vi "Command_Goto.vi"(2 "node":string, 3 "Side":T1, 4 "Desired Position":sgl=100.0 min=0 max=100, 6 "error in":errorcluster) -> (5 "error out":errorcluster)   [LabVIEW 2012]
doc: "This will open or close the gripper to a specific position"
uses:
  <userlib>/ROSforLV/ROS/Code/SubVIs/BaxterSide.ctl
  <userlib>/ROSforLV/ROS/Code/Console/Servers/ServerSubs/TopicDef.ctl
  <userlib>/ROSforLV/ROS/Code/SubVIs/_ROSDirection.ctl
panel:
  # "Gripper position is from [0.0-100.0] [close-open]"
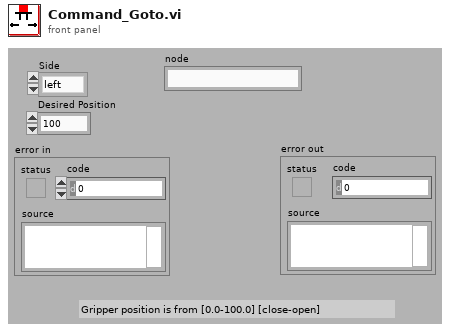
[diagram p1: front panel]
types:
  T1 = typedef "BaxterSide.ctl" = enum16{"left", "right"}
  T2 = typedef "TopicDef.ctl" = cluster{"Topic":string, "Type":string, "Action":T3, "Update (ms)":u16, "write queue":u16}
  T3 = typedef "_ROSDirection.ctl" = enum16{"Node", "Publisher", "Subscriber", "Service Client"}
  T4 = enum16{"no_op", "set", "configure", "reboot", "reset", "calibrate", "clear_calibration", "prepare_to_grip", "grip", "release", "go", "stop"}
  T5 = typedef "_ROSControl.ctl" = cluster{"topic port":u16, "Node":string, "topic":string, "type":string, "node port":u16, "error ":errorcluster, "Direction":T3, "APIs":string[], "Update (ms)":u16, "write queue":u16}
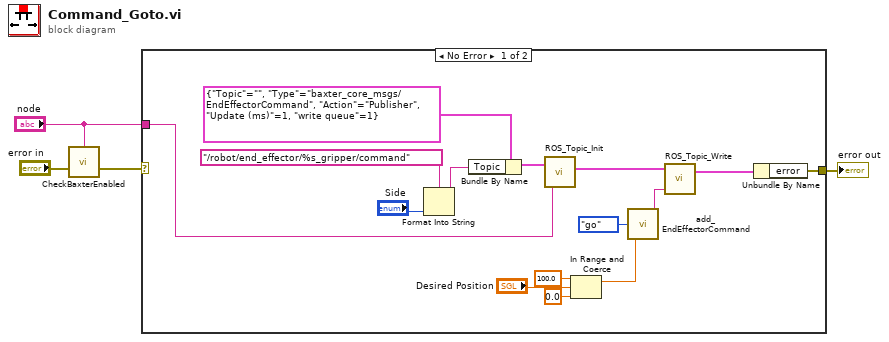
[diagram p0: block diagram]
diagram:
  n1 = call <userlib>:"CheckBaxterEnabled.vi"("error in"="error in", "node"="node") -> ("error out"=w2:errorcluster)  [unwired: 2 in]
  n2 = case shown="No Error" w2 {
    selector: w2 -> [_ w20]
    tunnel: [w17 w20] -> w4
    tunnel: "node" -> [w6 _]
    frame No Error {
      n3 = Format Into String(format string="/robot/end_effector/%s_gripper/command" ("Topic"), "Side") -> (resulting string=w9:string)  [unwired: 2 in, 1 out]
      n4 = Bundle By Name(cluster=T2 {"Topic"="", "Type"="baxter_core_msgs/EndEffectorCommand", "Action"=enum."Publisher", "Update (ms)"=1, "write queue"=1} ("Definitions"), "Topic"=w9) -> (w5:T2)
      n5 = call <userlib>:"ROS_Topic_Init.vi"("node"=w6, "Definitions"=w5) -> ("ROS out"=w19:T5)  [unwired: 1 in]
      n6 = In Range and Coerce(upper limit=sgl 100.0, x="Desired Position", lower limit=sgl 0.0) -> (coerced(x)=w12:sgl)  [unwired: 1 out]
      n7 = call <userlib>:"add_EndEffectorCommand.vi"("Position"=w12, "Commands"=T4."go") -> ("msg out"=w11:string)  [unwired: 3 in]
      n8 = call <userlib>:"ROS_Topic_Write.vi"("Msg in"=w11, "ROS in"=w19) -> ("ROS out"=w18:T5)  [unwired: 2 in]
      n9 = Unbundle By Name(w18) -> ("error"=w17:errorcluster)
    }
    frame Error {
    }
  }
  "error out" <- w4
